vi "UHR-Fleezers Control (host) - 10.4.vi"() -> ()   [LabVIEW 2011] (continued)
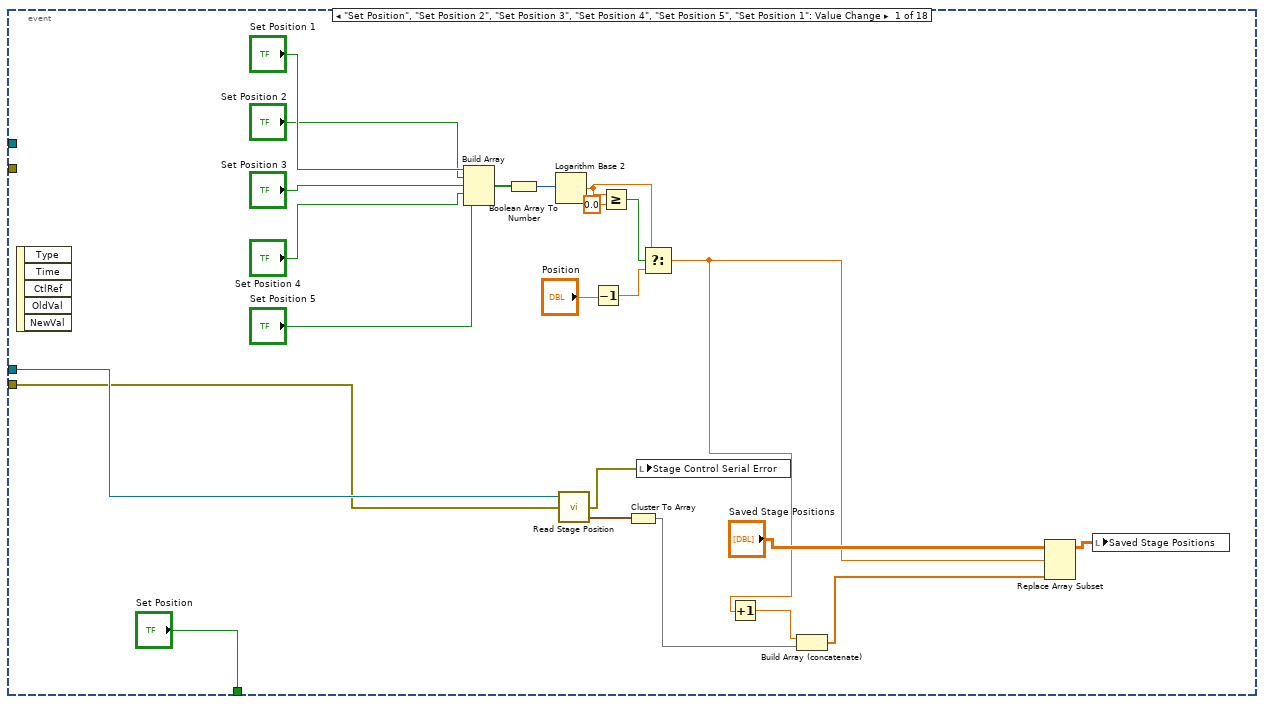
[diagram p2: hidden frame]
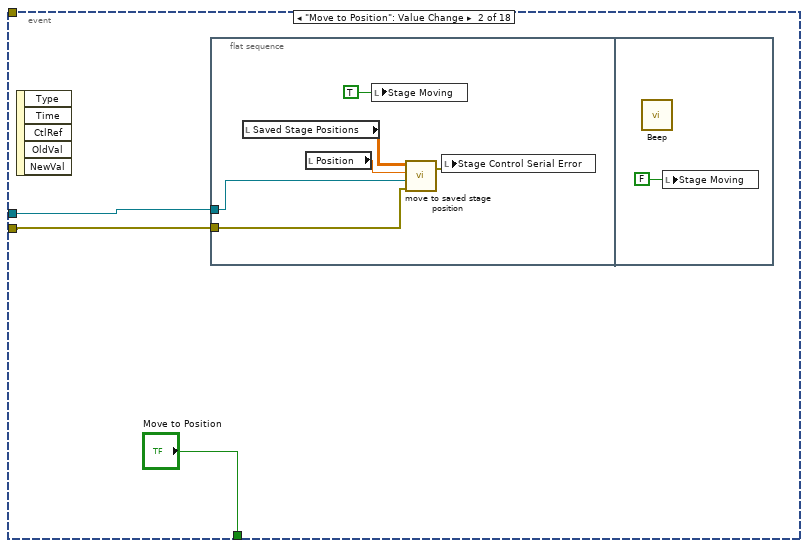
[diagram p3: hidden frame]
      tunnel: [w3040 w3060] -> w2741
      tunnel: [w3041 w3059] -> w2740
      frame False {
      }
      frame True {
        n2177 = xnode "Read/Write Control"("FPGA VI Reference In"=w3062, "error in"=w3061) -> ("FPGA VI Reference Out"=w3060:T19, "error out"=w3059:errorcluster, "GI Relative phase"=→"GI relative phase":i16, "Relative phase"=→"Relative phase (AI1)":i16, "AI Late Counter"=→"Late Counter (AI1)":u16, "GI Late Counter"=→"GI Late Counter":u16, "MCL Late Counter"=→"MCL Late Counter":u16, "MCL Relative Phase"=→"Relative Phase (MCL)":i16, "APD Acq Relative Phase"=→"APD Acq Relative Phase":i16, "APD 1 Gate Relative Phase"=→"APD 1 Gate Relative Phase":i16, "APD 2 Gate Relative Phase"=→"APD 2 Gate Relative Phase":i16, "APD Acq Late Counter"=→"APD Acq Late Counter":u16, "APD 1 Gate Late Counter"=→"APD 1 Gate Late Counter":u16, "APD 2 Gate Late Counter"=→"APD 2 Gate Late Counter":u16, "Green FB Relative Phase"=→"Relative phase (Green FB)":i16, "GI Relative phase 2"=→"GI relative phase 2":i16, "GI Late Counter 2"=→"GI Late Counter 2":u16, "Trap Pos FIFO Timeout"=→"Trap Pos FIFO Timeout":u16, "Trap AI FIFO Timeout"=→"Trap AI FIFO Timeout":u16)
      }
    }
    n2178 = call <vilib>:"Mean.vi"("X"=w2714) -> ("mean"=w2539:dbl)  [unwired: 1 out]
    "T2 X" <- w2539
    n2179 = Negate(x=w2714) -> (-x=w2715:dbl[])
    n2180 = call <vilib>:"Mean.vi"("X"=w2537) -> ("mean"=w2540:dbl)  [unwired: 1 out]
    "T1 X" <- w2540
    n2181 = Negate(x=w2539) -> (-x=w2538:dbl)
    n2182 = Bundle By Name(cluster=w2749, "Y"=w2712) -> (w2685:waveform(dbl))
    "Bead Separation" <- w2685
    n2183 = Add(x=w2537, y=w2715) -> (x+y=w2716:dbl[])
    n2184 = Add(x=w2540, y=w2538) -> (x+y=w2765:dbl)
    n2185 = Subtract(x=w2540, y=w2538) -> (x-y=→"Difference":dbl)
    n2186 = Divide(x=w2716, y=2.0) -> (x/y=→"Vec Mean of T1 T2":dbl[])
    n2187 = Divide(x=w2765, y=2.0) -> (x/y=w2718:dbl)
    "Mean" <- w2718
    n2188 = feedback-in #21("Trap Trig. Fl.") -> ()
    n2189 = feedback #21("Trap Trig. Fl.") -> (w2571:bool)
    n2190 = And(x=w2573, y=w2571) -> (x .and. y?=w2572:bool)
    n2191 = case "If have just turned off triggering" shown="True" w2572 {
      tunnel: w2553 -> [_ w2875]
      tunnel: w2552 -> [_ w2874]
      frame False {
      }
      frame True {
        w2873 = FALSE ("FPGA Trap Trig")
        n2192 = xnode "Read/Write Control"("FPGA VI Reference In"=w2875, "error in"=w2874, "FPGA Trap Trig"=w2873) -> ("FPGA VI Reference Out"=w2872:T19, "error out"=w2871:errorcluster)
        n2193 = xnode "Read/Write Control"("FPGA VI Reference In"=w2872, "error in"=w2871, "TTrig?"=w2873) -> ()  [unwired: 2 out]
        n2194 = local write "Initializing"(FALSE ("Initializing")) -> ()
        n2195 = local write "Triggered"(FALSE ("Triggered")) -> ()
        n2196 = local write "Waiting"(FALSE ("Waiting")) -> ()
      }
    }
    n2197 = Not(x=w2571) -> (.not. x?=w2584:bool)
    n2198 = And(x="Trap Trig. Fl.", y=w2584) -> (x .and. y?=w2581:bool)
    n2199 = local read "Tether"() -> (w2719:bool)
    n2200 = Or(x=w2581, y="Reinitialize") -> (x .or. y?=w2567:bool)
    n2201 = feedback #22(w2577) -> (w2582:string)
    n2202 = Select(t=w2577, s=w2581, f=w2582) -> (s? t:f=w2576:string)
    n2203 = Select(t=w2577, s="Reinitialize", f=w2576) -> (s? t:f=w2575:string)
    n2204 = feedback #23(0) -> (w2579:i32)
    n2205 = feedback #24(w2712) -> (w2711:dbl[])
    n2206 = Build Array (concatenate)(w2712, w2711) -> (w2710:dbl[])
    n2207 = case "For determining if there is a tether still" shown="True" w2719 {
      tunnel: w2718 -> [_ w2999]
      frame False {
      }
      frame True {
        n2208 = Greater?(x="Lost Tether Alarm Threshold (pN)", y=w2999) -> (0:w2997:bool)
        n2209 = case shown="True" w2997 {
          frame False {
          }
          frame True {
            w3000 = FALSE ("Value (Signaling)")
            n2210 = flat-sequence {
              frame #0 {
                # "stop only if saving"
                n2211 = local read "Saving..."() -> (w3012:bool)
                n2212 = And(x=w3012, y="TA Cancel Save?") -> (x .and. y?=w3011:bool)
                n2213 = local write "Stop Saving"(w3011) -> ()
              }
              frame #1 {
                n2214 = case shown="True" "TA Green Off?" {
                  frame False {
                  }
                  frame True {
                    w3015 = FALSE ("Fl. Triggered...")
                    n2215 = local write "Fl. Triggered..."(w3015) -> ()
                    n2216 = property on="Green Laser ON/Interlacing" class="Bool (strict)"("Val(Sgnl)"=w3015) -> ()  [unwired: 2 in, 2 out]
                  }
                }
              }
            }
            n2217 = local read "Time tether formed"() -> (w3006:timestamp)
            n2218 = Get Date/Time In Seconds() -> (seconds since 1Jan1904=w3007:timestamp)
            n2219 = Subtract(x=w3007, y=w3006) -> (x-y=w3005:dbl)
            n2220 = Number To Decimal String(number=w3005) -> (decimal integer string=w3002:string)  [unwired: 1 out]
            n2221 = local read "Messages"() -> (w3009:string)
            n2222 = call <vilib>:"Beep.vi"() -> ()  [unwired: 3 in, 9 out]
            n2223 = Concatenate Strings("Lost tether (" ("Message to add"), w3002, " s)." ("string")) -> (w3004:string)
            n2224 = local write "Tether"(FALSE ("Tether")) -> ()
            n2225 = call "Update messages.vi"("Message to add"=w3004, "Old message string"=w3009) -> ("New message string"=w3008:string)
            n2226 = local write "Messages"(w3008) -> ()
            n2227 = local write "Dip for Protein"(w3000) -> ()
            n2228 = property on="Trap Pos. FB ON" class="Bool (strict)"("Val(Sgnl)"=w3000) -> ()  [unwired: 2 in, 2 out]
            n2229 = property on="Trap Trig. Fl." class="Bool (strict)"("Val(Sgnl)"=w3000) -> ()  [unwired: 2 in, 2 out]
          }
        }
      }
    }
    n2230 = case "For triggering actions based on the trap position (e.g., turning the excitation laser on if trap under feedback moves so far)" shown="True" "Trap Trig. Fl." {
      tunnel: w2562 -> [_ w2888]
      tunnel: w2575 -> [_ w2887]
      tunnel: ["" ("t") w2886] -> w2583
      tunnel: w2567 -> [_ w2885]
      tunnel: [0 ("t") w2884] -> w2580
      tunnel: w2579 -> [_ w2883]
      tunnel: w2553 -> [_ w2882]
      tunnel: w2552 -> [_ w2881]
      frame False {
      }
      frame True {
        n2231 = case shown="\"Initialize\", Default" w2887 {
          tunnel: w2888 -> [w2905 _ _ w2953]
          tunnel: [w2902 w2934 "" ("t") w2956] -> w2886
          tunnel: w2885 -> [_ _ _ w2944]
          tunnel: [w2901 w2931 0 ("t") w2945] -> w2884
          tunnel: w2883 -> [_ w2933 _ w2951]
          tunnel: w2882 -> [w2890 w2928 _ w2947]
          tunnel: w2881 -> [w2889 w2927 _ w2946]
          frame "Wait for trigger" {
            n2232 = local read "Trap Trig. (FPGA)"() -> (w2893:bool)
            n2233 = Subtract(x=w2905, y="Mean T1 Position\nto compare (nm)") -> (x-y=w2898:dbl[])
            n2234 = call <vilib>:"Std Deviation and Variance.vi"("X"=w2898) -> ("mean"=→"mean":dbl, "standard deviation"=→"standard\ndeviation":dbl)  [unwired: 1 in, 1 out]
            n2235 = Array Max & Min(array=w2898) -> (max value=→"max value":dbl, min value=→"min value":dbl)  [unwired: 2 out]
            n2236 = Greater?(x=w2898, y="Threshold (nm)") -> (0:w2908:bool[])
            n2237 = case shown="True" w2893 {
              tunnel: w2890 -> [_ w2914]
              tunnel: w2889 -> [_ w2913]
              tunnel: [FALSE ("TTrig?") w2912] -> w2896
              frame False {
              }
              frame True {
                n2238 = xnode "Read/Write Control"("FPGA VI Reference In"=w2914, "error in"=w2913) -> ("TTrig?"=w2912:bool)  [unwired: 2 out]
              }
            }
            n2239 = Or Array Elements(Boolean array=w2908) -> (logical OR=w2895:bool)
            n2240 = Select(t=w2896, s=w2893, f=w2895) -> (s? t:f=w2894:bool)
            n2241 = Not(x=w2893) -> (.not. x?=w2892:bool)
            n2242 = And(x=w2894, y=w2892) -> (x .and. y?=w2891:bool)
            n2243 = Select(t="Triggered", s=w2894, f="Wait for trigger") -> (s? t:f=w2902:string)
            n2244 = case shown="True" w2894 {
              tunnel: [0 0] -> w2901
              tunnel: w2890 -> [_ w2919]
              tunnel: w2889 -> [_ w2918]
              frame False {
                "Waiting" <- TRUE ("Waiting")
              }
              frame True {
                n2245 = xnode "Read/Write Control"("FPGA VI Reference In"=w2919, "error in"=w2918, "TTrig?"=FALSE) -> ()  [unwired: 2 out]
                n2246 = local read "Messages"() -> (w2922:string)
                n2247 = call <vilib>:"Beep.vi"() -> ()  [unwired: 12 in]
                n2248 = call "Update messages.vi"("Message to add"="Unwinding trigger.", "Old message string"=w2922) -> ("New message string"=w2923:string)
                n2249 = local write "Messages"(w2923) -> ()
                n2250 = local write "Waiting"(FALSE ("Waiting")) -> ()
                "Triggered" <- TRUE ("Triggered")
              }
            }
            n2251 = case "Only need to turn on laser if host triggered" shown="True" w2891 {
              frame False {
              }
              frame True {
                n2252 = property on="Green Laser ON/Interlacing" class="Bool (strict)"("Val(Sgnl)"=TRUE ("Value (Signaling)")) -> ()  [unwired: 2 in, 2 out]
              }
            }
          }
          frame "Triggered" {
            n2253 = local read "Trap Trig. (FPGA)"() -> (w2930:bool)
            n2254 = Increment(x=w2933) -> (x+1=w2931:i32)
            n2255 = Greater Or Equal?(x=w2931, y="Fl. ON time (n)") -> (x >= y?=w2929:bool)
            n2256 = Select(t="Wait for trigger", s=w2929, f="Triggered" ("t")) -> (s? t:f=w2934:string)
            n2257 = And(x=w2929, y=w2930) -> (x .and. y?=w2926:bool)
            n2258 = case shown="True" w2926 {
              tunnel: w2928 -> [_ w2938]
              tunnel: w2927 -> [_ w2937]
              frame False {
              }
              frame True {
                n2259 = xnode "Read/Write Control"("FPGA VI Reference In"=w2938, "error in"=w2937, "FPGA Trap Trig"=TRUE) -> ()  [unwired: 2 out]
              }
            }
            n2260 = case shown="True" w2929 {
              frame False {
              }
              frame True {
                w2940 = FALSE ("Value (Signaling)")
                n2261 = local write "Triggered"(w2940) -> ()
                n2262 = local write "Waiting"(TRUE ("Waiting")) -> ()
                n2263 = property on="Green Laser ON/Interlacing" class="Bool (strict)"("Val(Sgnl)"=w2940) -> ()  [unwired: 2 in, 2 out]
              }
            }
          }
          frame "Do nothing" {
          }
          frame "Initialize", Default {
            n2264 = Increment(x=w2951) -> (x+1=w2955:i32)
            n2265 = Select(t=1, s=w2944, f=w2955) -> (s? t:f=w2945:i32)
            n2266 = feedback #25(w2953) -> (w2959:dbl[])
            n2267 = Build Array (concatenate)(w2953, w2959) -> (w2952:dbl[])
            n2268 = Greater Or Equal?(x=w2945, y="Wait to get offset (n)") -> (x >= y?=w2948:bool)
            n2269 = Select(t=w2953, s=w2944, f=w2952) -> (s? t:f=w2954:dbl[])
            n2270 = feedback-in #25(w2954) -> ()
            n2271 = call <vilib>:"Mean.vi"("X"=w2954) -> ("mean"=w2949:dbl)  [unwired: 1 out]
            n2272 = local write "Mean T1 Position\nto compare (nm)"(w2949) -> ()
            n2273 = case shown="True" w2944 {
              tunnel: w2947 -> [_ w2965]
              tunnel: w2946 -> [_ w2964]
              frame False {
              }
              frame True {
                w2961 = FALSE ("FPGA Trap Trig")
                n2274 = xnode "Read/Write Control"("FPGA VI Reference In"=w2965, "error in"=w2964, "FPGA Trap Trig"=w2961) -> ("FPGA VI Reference Out"=w2963:T19, "error out"=w2962:errorcluster)
                n2275 = xnode "Read/Write Control"("FPGA VI Reference In"=w2963, "error in"=w2962, "TTrig?"=w2961) -> ()  [unwired: 2 out]
              }
            }
            n2276 = Select(t="Wait for trigger", s=w2948, f="Initialize") -> (s? t:f=w2956:string)
            n2277 = case shown="True" w2948 {
              tunnel: w2949 -> [_ w2968]
              tunnel: w2947 -> [_ w2977]
              tunnel: w2946 -> [_ w2976]
              frame False {
                n2278 = local write "Waiting"(FALSE ("Waiting")) -> ()
                "Initializing" <- TRUE ("Initializing")
              }
              frame True {
                n2279 = local read "Threshold (nm)"() -> (w2980:dbl)
                n2280 = local read "AOM X Cal (nm/MHz)"() -> (w2979:dbl)
                n2281 = Add(x=w2968, y=w2980) -> (x+y=w2981:dbl)
                n2282 = Divide(x=w2981, y=w2979) -> (x/y=w2978:dbl)
                n2283 = call "IR AOM freq to word.vi"("Frequency In (MHz)"=w2978) -> ("Frequency Word Out (double)"=w2975:dbl)
                n2284 = local write "Initializing"(FALSE ("Initializing")) -> ()
                n2285 = local write "Waiting"(TRUE ("Waiting")) -> ()
                n2286 = To Quad Integer(1:w2975) -> (0:w2974:i64)
                n2287 = xnode "Read/Write Control"("FPGA VI Reference In"=w2977, "error in"=w2976, "FPGA TTrig Thresh"=w2974) -> ("FPGA VI Reference Out"=w2971:T19, "error out"=w2970:errorcluster)
                n2288 = xnode "Read/Write Control"("FPGA VI Reference In"=w2971, "error in"=w2970, "FPGA Trap Trig"=TRUE) -> ()  [unwired: 2 out]
              }
            }
          }
        }
      }
    }
    n2289 = feedback-in #22(w2583) -> ()
    n2290 = feedback-in #23(w2580) -> ()
    n2291 = Split 1D Array(array=w2710, index=w2597) -> (first subarray=w2707:dbl[])  [unwired: 1 out]
    n2292 = feedback-in #24(w2707) -> ()
    n2293 = call <vilib>:"Mean.vi"("X"=w2707) -> ("mean"=w2706:dbl)  [unwired: 1 out]
    "Bead Mean (nm)" <- w2706
    n2294 = Subtract(x=w2707, y=w2706) -> (x-y=w2705:dbl[])
    n2295 = Square(x=w2705) -> (x^2=w2704:dbl[])
    n2296 = call <vilib>:"Mean.vi"("X"=w2704) -> ("mean"=w2703:dbl)  [unwired: 1 out]
    n2297 = Square Root(x=w2703) -> (sqrt(x)=w2702:dbl)
    n2298 = Multiply(x=10.0, y=w2702) -> (x*y=→"RMS (Ang)":dbl)
    n2299 = xnode "Read/Write Control"("FPGA VI Reference In"=w2741, "error in"=w2740) -> ("FPGA VI Reference Out"=w2565:T19, "error out"=w2564:errorcluster, "AI2 Y Sum Set 1"=w2849:i16, "AI2 Y Sum Set 2"=w2848:i16, "AI1 X Set 1"=w2629:fxp<+/-,16,1>, "AI1 X Set 2"=w2628:fxp<+/-,16,1>, "Trap Pos FB Int Signal"=→"Trap Pos FB Int Signal":fxp<+/-,24,9>, "Trap Pos FB Int-Norm Signal"=→"Trap Pos FB Int-Norm Signal":fxp<+/-,16,1>, "Trap Pos FB Action"=w2622:i64, "Scanning"=→"AOD Scanning":bool, "Scan I"=→"AOD Scan I":u64, "Scanning MCL"=w2851:bool, "Scan I (MCL)"=→"MCL Scan I":u64, "Green FB Signals"=w2788:T46, "TTrig Sig"=w2551:i64, "TTrig Fin Thresh"=w2547:i64)
    "MCL Scanning" <- w2851
    "Trap Pos FB Action" <- w2622
    n2300 = local read "FB Trig Integrate"() -> (w2545:u32)
    n2301 = Divide(x=w2551, y=w2545) -> (x/y=w2544:dbl)
    "TTrig Sig (Int)" <- w2544
    n2302 = Divide(x=w2547, y=w2545) -> (x/y=w2542:dbl)
    "TTrig Fin Thresh (Int)" <- w2542
    n2303 = local read "AOM X Cal (nm/MHz)"() -> (w2550:dbl)
    n2304 = local read "AI2 (V)"() -> (w2850:cluster{"Set 1":dbl, "Set 2":dbl})
    n2305 = Bundle By Name(cluster=w2850, "Set 1"=w2849, "Set 2"=w2848) -> (w2846:cluster{"Set 1":dbl, "Set 2":dbl})
    n2306 = Divide(x=w2622, y=327.67) -> (x/y=→"Action (%)":dbl)
    n2307 = local read "Trap X (AI1)"() -> (w2642:T10)
    n2308 = call "IR AOM word double to freq.vi"("Frequency Word In (double)"=w2542) -> ("Frequency Out (MHz)"=w2541:dbl)
    n2309 = call "IR AOM word double to freq.vi"("Frequency Word In (double)"=w2544) -> ("Frequency Out (MHz)"=w2543:dbl)
    n2310 = Divide(x=w2846, y=3276.7) -> (x/y=w2845:cluster{"Set 1":dbl, "Set 2":dbl})
    n2311 = Multiply(x=w2543, y=w2550) -> (x*y=w2549:dbl)
    "TTrig Sig (nm)" <- w2549
    n2312 = Multiply(x=w2541, y=w2550) -> (x*y=w2548:dbl)
    "TTrig Fin Thresh (nm)" <- w2548
    n2313 = local write "AI2 (V)"(w2845) -> ()
    n2314 = Bundle(cluster=w2642, "Trap 1"=w2629, "Trap 2"=w2628) -> (→"Trap X (AI1)":T10)
    n2315 = Bundle(w2549, w2548) -> (→"TTrig":cluster{dbl, dbl})  [unwired: 1 in]
    n2316 = Divide(x=w2788, y=3276.7) -> (x/y=w2784:T47)
    n2317 = Unbundle By Name(w2784) -> ("Green FB Ch 0"=w2787:dbl, "Green FB Ch 1"=w2786:dbl, "Green FB Ch 2"=w2785:dbl)
    n2318 = Divide(x=w2787, y=w2785) -> (x/y=w2783:dbl)
    n2319 = Divide(x=w2786, y=w2785) -> (x/y=w2782:dbl)
    n2320 = flat-sequence "To save data" {
      tunnel: [w3836] -> w2869
      tunnel: [w3837] -> w2868
      tunnel: w2819 -> [w3830]
      tunnel: w2570 -> [w3834]
      tunnel: ["Save Calibration"] -> w2842
      tunnel: w2839 -> [w3833]
      tunnel: [w3826] -> w2838
      tunnel: [w3823] -> w2837
      tunnel: [w3820] -> w2836
      tunnel: w2818 -> [w3822]
      tunnel: w2723 -> [w3816]
      tunnel: [w3816] -> w2722
      tunnel: ["Start Saving"] -> w2687
      tunnel: [w3810] -> w2610
      tunnel: [w3809] -> w2609
      tunnel: w2869 -> [w4071]
      tunnel: w2868 -> [w4070]
      tunnel: w2611 -> [w4069]
      tunnel: w2842 -> [w4068]
      tunnel: w2838 -> [w4066]
      tunnel: w2837 -> [w4065]
      tunnel: w2836 -> [w4064]
      tunnel: w2696 -> [w4063]
      tunnel: w2733 -> [w4062]
      tunnel: w2722 -> [w4061]
      tunnel: w2687 -> [w4060]
      tunnel: w2685 -> [w4059]
      tunnel: w2661 -> [w4058]
      tunnel: w2610 -> [w4057]
      tunnel: w2609 -> [w4056]
      tunnel: w2608 -> [w4055]
      frame #0 {
        n2321 = Or(x="Save N Sets", y="Start Saving") -> (x .or. y?=w3817:bool)
        n2322 = To Double Precision Float(number=w3833) -> (double precision float=w3827:dbl)
        n2323 = Build Array(w3817, "Save Calibration", w3830, w3822) -> (w3832:bool[])
        n2324 = Compound Arithmetic op=OR("Save Calibration", w3830, w3817, w3822) -> (w3835:bool)
        n2325 = Boolean Array To Number(Boolean array=w3832) -> (number=w3829:u32)
        n2326 = feedback #26(FALSE ("Save APD Data\nwith Trap Data")) -> (w3811:bool)
        n2327 = feedback #27(refnum<k0> refnum) -> (w3838:refnum<file>)
        n2328 = feedback #28(refnum<k0> refnum) -> (w3813:refnum<file>)
        n2329 = feedback #29(FALSE ("Save APD Data\nwith Trap Data")) -> (w3821:bool)
        n2330 = feedback #30(refnum<k0> refnum) -> (w3824:refnum<file>)
        n2331 = feedback #31(0) -> (w3840:i32)
        n2332 = feedback #32() -> (w3828:u32)  [unwired: 1 out]
        n2333 = case shown="True" w3835 {
          tunnel: [w3847 1] -> w3836
          tunnel: w3840 -> [w3849 _]
          tunnel: [w3848 w3867] -> w3837
          tunnel: w3838 -> [w3848 _]
          tunnel: w3834 -> [_ w3887]
          tunnel: w3827 -> [_ w3885]
          tunnel: w3829 -> [_ w3888]
          tunnel: [w3846 w3866] -> w3826
          tunnel: w3828 -> [w3846 _]
          tunnel: [w3845 w3864] -> w3823
          tunnel: w3824 -> [w3845 _]
          tunnel: [w3844 w3863] -> w3820
          tunnel: w3821 -> [w3844 _]
          tunnel: "Start Saving" -> [_ w3861]
          tunnel: w3816 -> [_ w3860]
          tunnel: [w3843 w3851] -> w3809
          tunnel: w3813 -> [w3843 _]
          tunnel: [w3842 w3850] -> w3810
          tunnel: w3811 -> [w3842 _]
          frame False {
            n2334 = Increment(x=w3849) -> (x+1=w3847:i32)
          }
          frame True {
            w3857 = FALSE ("Start Saving")
            w3862 = 9.0  # File Version
            w3870 = FALSE ("prepend array or string size? (T)")
            w3868 = T24."big-endian, network order" ("byte order (0:big-endian, network order)")
            n2335 = local read "BD 1 Frequency 1 (MHz)"() -> (w3884:dbl)
            n2336 = local read "BD 2 Frequency 1 (MHz)"() -> (w3883:dbl)
            n2337 = local read "BD 1 Frequency 2 (MHz)"() -> (w3882:dbl)
            n2338 = local read "BD 2 Frequency 2 (MHz)"() -> (w3881:dbl)
            n2339 = local read "BD 1 Frequency 3 (MHz)"() -> (w3880:dbl)
            n2340 = local read "BD 2 Frequency 3 (MHz)"() -> (w3879:dbl)
            n2341 = Array Size(array=w3860) -> (size(s)=w3859:i32)
            n2342 = To Double Precision Float(number=w3859) -> (double precision float=w3858:dbl)
            n2343 = local write "Save Calibration"(w3857) -> ()
            n2344 = local write "Start Saving"(w3857) -> ()
            n2345 = Build Array("Save APD Data\nwith Trap Data", "Save Trap Pos. Data") -> (w3854:bool[])
            n2346 = Boolean Array To Number(Boolean array=w3854) -> (number=w3853:u32)
            n2347 = Build Array(w3884, w3883, w3882, w3881, w3880, w3879) -> (w3878:dbl[])
            n2348 = case shown="4" w3888 {
              tunnel: w3887 -> [w3959 w3979 w3995 w4033]
              tunnel: w3858 -> [w3964 w3986 w4015 w4052]
              tunnel: w3885 -> [w3963 w3985 w4014 w4051]
              tunnel: [w3960 w3981 w4006 w4043] -> w3876
              tunnel: [w3951 "Cal sets to save" w3996 w4034] -> w3866
              tunnel: w3878 -> [w3961 w3982 w4008 w4045]
              tunnel: "Save APD Data\nwith Trap Data" -> [w3958 _ w3992 w4031]
              tunnel: [w3958 w3973 w3992 w4031] -> w3863
              tunnel: w3862 -> [w3954 w3974 w3990 w4029]
              tunnel: w3861 -> [w3953 _ _ _]
              tunnel: [w3944 w3973 w3989 w4019] -> w3850
              tunnel: "Save Trap Pos. Data" -> [w3944 _ w3989 w4019]
              tunnel: w3853 -> [w3943 _ w3988 w4018]
              frame 1, Default {
                # "timeseries"
                n2349 = case shown="True" "Profile" {
                  tunnel: [w3967 w3971] -> w3948
                  tunnel: [w3967 w3970] -> w3947
                  tunnel: [w3967 w3969] -> w3946
                  tunnel: [w3967 w3968] -> w3945
                  frame False {
                    w3967 = 0.0 ("f")
                  }
                  frame True {
                    n2350 = local read "Current Position"() -> (w3972:cluster{dbl, dbl, dbl})
                    n2351 = local read "Y change (mm)"() -> (w3968:dbl)
                    n2352 = Unbundle(w3972) -> (w3971:dbl, w3970:dbl, w3969:dbl)
                  }
                }
                n2353 = local read "Save ave N"() -> (w3966:dbl)
                n2354 = Multiply(x=w3966, y=w3959) -> (x*y=w3965:dbl)
                n2355 = To Double Precision Float(number=w3943) -> (double precision float=w3957:dbl)
                n2356 = Build Array(w3954, w3959, w3965, w3964, w3963, 0.0 ("f")) -> (w3962:dbl[])
                n2357 = Build Array(w3957, w3948, w3947, w3946, w3945) -> (w3955:dbl[])
                n2358 = Select(t=u32 4000000000, s=w3953, f="N sets to save") -> (s? t:f=w3951:u32)
                n2359 = Build Array (concatenate)(w3962, w3961, w3955) -> (w3960:dbl[])
              }
              frame 2 {
                w3976 = 0.0 ("f")
                w3973 = FALSE ("Save APD Data\nwith Trap Data")
                # "calibration"
                n2360 = Boolean To (0,1)(Boolean=w3973) -> (0, 1=w3978:i16)
                n2361 = To Double Precision Float(number=w3978) -> (double precision float=w3977:dbl)
                n2362 = Build Array(w3977, w3976, w3976, w3976, w3976) -> (w3975:dbl[])
                n2363 = Build Array(w3974, w3979, w3979, w3986, w3985, 1.0 ("t")) -> (w3983:dbl[])
                n2364 = Build Array (concatenate)(w3983, w3982, w3975) -> (w3981:dbl[])
                "Calibrating Trap..." <- TRUE ("Calibrating...")
              }
              frame 4 {
                w3993 = 0.0 ("f")
                # "scan dir (x/y = 0/1)"
                # "cycles/step"
                # "n scans (f/b)"
                # "steps"
                # "freq. range"
                # "AOD raster scan"
                n2365 = local read "Number of F/B Scans (AOD)"() -> (w4000:u16)
                n2366 = local read "Cycles/step (AOD)"() -> (w4002:u64)
                n2367 = local read "Scan Range (MHz)"() -> (w4005:dbl)
                n2368 = local read "Scan steps (AOD)"() -> (w4004:u64)
                n2369 = local read "Scan BD"() -> (w4012:bool)
                n2370 = local read "Save ave N"() -> (w4017:dbl)
                n2371 = Boolean To (0,1)(Boolean=w4012) -> (0, 1=w4011:i16)
                n2372 = To Double Precision Float(number=w4000) -> (double precision float=w3999:dbl)
                n2373 = To Double Precision Float(number=w4004) -> (double precision float=w4003:dbl)
                n2374 = To Double Precision Float(number=w4002) -> (double precision float=w4001:dbl)
                n2375 = To Double Precision Float(number=w4011) -> (double precision float=w4010:dbl)
                n2376 = Multiply(x=w4017, y=w3995) -> (x*y=w4016:dbl)
                n2377 = To Double Precision Float(number=w3988) -> (double precision float=w3994:dbl)
                n2378 = Build Array(w3994, w3993, w3993, w3993, w3993) -> (w3991:dbl[])
                n2379 = local read "N sets should be saved"() -> (w3997:dbl)
                n2380 = Build Array(w4010, w4005, w4003, w4001, w3999) -> (w4007:dbl[])
                n2381 = Build Array(w3990, w3995, w4016, w4015, w4014, 2.0 ("t")) -> (w4009:dbl[])
                n2382 = Round Toward +Infinity(x=w3997) -> (ceil(x): smallest int >= x=w3998:dbl)
                n2383 = Build Array (concatenate)(w4009, w4008, w3991, w4007) -> (w4006:dbl[])
                n2384 = To Unsigned Long Integer(number=w3998) -> (unsigned 32bit integer=w3996:u32)
              }
              frame 8 {
                w4026 = 0.0 ("f")
                # "MCL raster scan"
                n2385 = local read "Number of scans (MCL)"() -> (w4021:u64)
                n2386 = local read "Scan lines (y)"() -> (w4020:u64)
                n2387 = local read "2D or 1D Scan"() -> (w4023:bool)
                n2388 = local read "Scan Range (V)\n(of steps)"() -> (w4042:dbl)
                n2389 = local read "Fast Scan Dir"() -> (w4049:bool)
                n2390 = local read "Cycles/step (MCL)"() -> (w4039:u64)
                n2391 = local read "Scan steps (MCL)"() -> (w4041:u64)
                n2392 = Select(t=w4020, s=w4023, f=w4021) -> (s? t:f=w4022:u64)
                n2393 = Boolean To (0,1)(Boolean=w4023) -> (0, 1=w4025:i16)
                n2394 = local read "Save ave N"() -> (w4054:dbl)
                n2395 = local read "Initial X"() -> (w4028:dbl)
                n2396 = local read "Initial Y"() -> (w4027:dbl)
                n2397 = To Double Precision Float(number=w4025) -> (double precision float=w4024:dbl)
                n2398 = Boolean To (0,1)(Boolean=w4049) -> (0, 1=w4048:i16)
                n2399 = To Double Precision Float(number=w4022) -> (double precision float=w4037:dbl)
                n2400 = To Double Precision Float(number=w4041) -> (double precision float=w4040:dbl)
                n2401 = To Double Precision Float(number=w4039) -> (double precision float=w4038:dbl)
                n2402 = To Double Precision Float(number=w4048) -> (double precision float=w4047:dbl)
                n2403 = Multiply(x=w4054, y=w4033) -> (x*y=w4053:dbl)
                n2404 = To Double Precision Float(number=w4018) -> (double precision float=w4032:dbl)
                n2405 = local read "N sets should be saved (MCL)"() -> (w4035:dbl)
                n2406 = Build Array(w4032, w4024, w4026, w4026, w4026) -> (w4030:dbl[])
                n2407 = Build Array(w4047, w4042, w4040, w4038, w4037, w4028, w4027) -> (w4044:dbl[])
                n2408 = Build Array(w4029, w4033, w4053, w4052, w4051, 3.0 ("t")) -> (w4046:dbl[])
                n2409 = Round Toward +Infinity(x=w4035) -> (ceil(x): smallest int >= x=w4036:dbl)
                n2410 = Build Array (concatenate)(w4046, w4045, w4030, w4044) -> (w4043:dbl[])
                n2411 = To Unsigned Long Integer(number=w4036) -> (unsigned 32bit integer=w4034:u32)
              }
            }
            n2412 = local read "Index"() -> (w3893:dbl)
            n2413 = call "Create new save file.vi"("Insert"="", "Ext"=".dat", "Index In"=w3893) -> ("Path Out"=w3852:path, "Index Out"=w3865:dbl)
            n2414 = local write "Save file name"(w3852) -> ()
            n2415 = local write "Index"(w3865) -> ()
            n2416 = local write "Save index"(w3865) -> ()
            n2417 = Array Size(array=w3876) -> (size(s)=w3877:i32)
            n2418 = Open/Create/Replace File(file path (use dialog)=w3852, operation (0:open)=T25."create", access (0:read/write)=enum16{"read/write", "read-only", "write-only"}."write-only") -> (refnum out=w3890:refnum<file>)  [unwired: 1 in, 4 out]
            n2419 = local write "Saving..."(TRUE ("Saving...")) -> ()
            n2420 = To Double Precision Float(number=w3877) -> (double precision float=w3875:dbl)
            n2421 = String Length(string="Comment (data description)") -> (length=w3873:i32)
            n2422 = To Double Precision Float(number=w3873) -> (double precision float=w3872:dbl)
            n2423 = Deny Access(7:w3890) -> (3:w3889:refnum<file>)  [unwired: 1 in, 2 out]
            n2424 = Build Array (concatenate)(w3875, w3876, w3872) -> (w3874:dbl[])
            n2425 = case "If fluorescence data to be saved" shown="True" w3863 {
              tunnel: w3852 -> [_ w3942]
              tunnel: [refnum<k0> refnum w3922] -> w3864
              frame False {
              }
              frame True {
                w3921 = 0.0
                n2426 = local read "APD Integration Time (s)"() -> (w3927:dbl)
                n2427 = local read "N APD Samp/step"() -> (w3920:dbl)
                n2428 = Path To String(path=w3942) -> (string=w3941:string)
                n2429 = String Length(string=w3941) -> (length=w3940:i32)
                n2430 = Subtract(x=w3940, y=4) -> (x-y=w3938:i32)
                n2431 = String Subset(string=w3941, length (rest)=w3938) -> (substring=w3937:string)  [unwired: 1 out]
                n2432 = Build Array(w3927, w3920, w3921, w3921, w3921, w3921, w3921, w3921) -> (w3924:dbl[])
                n2433 = Concatenate Strings(w3937, "_fl.dat" ("string")) -> (w3935:string)
                n2434 = Array Size(array=w3924) -> (size(s)=w3926:i32)
                n2435 = String To Path(string=w3935) -> (path=w3931:path)
                n2436 = Open/Create/Replace File(file path (use dialog)=w3931, operation (0:open)=T25."create", access (0:read/write)=enum16{"read/write", "read-only", "write-only"}."write-only") -> (refnum out=w3932:refnum<file>)  [unwired: 1 in, 4 out]
                n2437 = Deny Access(7:w3932) -> (3:w3928:refnum<file>)  [unwired: 1 in, 2 out]
                n2438 = To Double Precision Float(number=w3926) -> (double precision float=w3925:dbl)
                n2439 = Build Array (concatenate)(w3925, w3924) -> (w3923:dbl[])
                n2440 = Write to Binary File(file (use dialog)=w3928, data=w3923, 5:FALSE ("prepend array or string size? (T)"), 9:T24."big-endian, network order" ("byte order (0:big-endian, network order)")) -> (refnum out=w3922:refnum<file>)  [unwired: 1 in, 3 out]
              }
            }
            n2441 = case shown="True" w3850 {
              tunnel: w3852 -> [_ w3904]
              tunnel: [refnum<k0> refnum w3903] -> w3851
              frame False {
              }
              frame True {
                w3899 = 0.0 ("element")
                n2442 = Path To String(path=w3904) -> (string=w3918:string)
                n2443 = Build Array(w3899, w3899, w3899, w3899, w3899, w3899, w3899, w3899) -> (w3900:dbl[])
                n2444 = String Length(string=w3918) -> (length=w3917:i32)
                n2445 = Subtract(x=w3917, y=4) -> (x-y=w3915:i32)
                n2446 = Array Size(array=w3900) -> (size(s)=w3902:i32)
                n2447 = String Subset(string=w3918, length (rest)=w3915) -> (substring=w3914:string)  [unwired: 1 out]
                n2448 = To Double Precision Float(number=w3902) -> (double precision float=w3901:dbl)
                n2449 = Concatenate Strings(w3914, "_pos.dat" ("string")) -> (w3912:string)
                n2450 = Build Array (concatenate)(w3901, w3900) -> (w3898:dbl[])
                n2451 = String To Path(string=w3912) -> (path=w3908:path)
                n2452 = Open/Create/Replace File(file path (use dialog)=w3908, operation (0:open)=T25."create", access (0:read/write)=enum16{"read/write", "read-only", "write-only"}."write-only") -> (refnum out=w3909:refnum<file>)  [unwired: 1 in, 4 out]
                n2453 = Deny Access(7:w3909) -> (3:w3905:refnum<file>)  [unwired: 1 in, 2 out]
                n2454 = Write to Binary File(file (use dialog)=w3905, data=w3898, 5:FALSE ("prepend array or string size? (T)"), 9:T24."big-endian, network order" ("byte order (0:big-endian, network order)")) -> (refnum out=w3903:refnum<file>)  [unwired: 1 in, 3 out]
              }
            }
            n2455 = Write to Binary File(file (use dialog)=w3889, data=w3874, 5:w3870, 9:w3868) -> (refnum out=w3871:refnum<file>)  [unwired: 1 in, 3 out]
            n2456 = Write to Binary File(file (use dialog)=w3871, data="Comment (data description)", 5:w3870, 9:w3868) -> (refnum out=w3867:refnum<file>)  [unwired: 1 in, 3 out]
          }
        }
        n2457 = feedback-in #26(w3810) -> ()
        n2458 = feedback-in #27(w3837) -> ()
        n2459 = feedback-in #28(w3809) -> ()
        n2460 = feedback-in #29(w3820) -> ()
        n2461 = feedback-in #30(w3823) -> ()
        n2462 = feedback-in #31(w3836) -> ()
        n2463 = feedback-in #32(w3826) -> ()
      }
      frame #1 {
        n2464 = local read "Saving..."() -> (w4067:bool)
        n2465 = case shown="True" w4067 {
          tunnel: w4071 -> [_ w4081]
          tunnel: w4070 -> [_ w4095]
          tunnel: w4069 -> [_ w4091]
          tunnel: w4068 -> [_ w4090]
          tunnel: w4066 -> [_ w4089]
          tunnel: w4065 -> [_ w4084]
          tunnel: w4064 -> [_ w4083]
          tunnel: w4063 -> [_ w4082]
          tunnel: w4062 -> [_ w4080]
          tunnel: w4061 -> [_ w4078]
          tunnel: w4060 -> [_ w4077]
          tunnel: w4059 -> [_ w4076]
          tunnel: w4058 -> [_ w4075]
          tunnel: w4057 -> [_ w4074]
          tunnel: w4056 -> [_ w4073]
          tunnel: w4055 -> [_ w4072]
          frame False {
          }
          frame True {
            n2466 = Multiply(x=w4081, y=w4080) -> (x*y=→"Time (s)":dbl)
            n2467 = Less Or Equal?(x=w4081, y=w4089) -> (x <= y?=w4093:bool)
            n2468 = Or(x="Stop Saving", y="Abort save 2") -> (x .or. y?=w4085:bool)
            n2469 = Not(x=w4085) -> (.not. x?=w4094:bool)
            n2470 = And(x=w4093, y=w4094) -> (x .and. y?=w4092:bool)
            n2471 = case shown="True" w4092 {
              tunnel: w4095 -> [w4102 w4170]
              tunnel: [0.0 w4173] -> w4088
              tunnel: w4081 -> [_ w4171]
              tunnel: w4089 -> [_ w4172]
              tunnel: w4091 -> [_ w4167]
              tunnel: w4090 -> [_ _]
              tunnel: w4084 -> [w4100 w4160]
              tunnel: w4083 -> [w4099 w4161]
              tunnel: w4082 -> [_ w4159]
              tunnel: w4078 -> [_ w4158]
              tunnel: w4077 -> [_ w4112]
              tunnel: w4076 -> [_ w4151]
              tunnel: w4075 -> [_ w4129]
              tunnel: w4074 -> [w4096 w4110]
              tunnel: w4073 -> [w4097 w4109]
              tunnel: w4072 -> [_ w4106]
              frame False {
                w4098 = FALSE
                n2472 = Close File(refnum=w4102) -> ()  [unwired: 1 in, 2 out]
                n2473 = case shown="True" w4099 {
                  tunnel: w4100 -> [_ w4104]
                  frame False {
                  }
                  frame True {
                    n2474 = Close File(refnum=w4104) -> ()  [unwired: 1 in, 2 out]
                  }
                }
                n2475 = case shown="True" w4096 {
                  tunnel: w4097 -> [_ w4103]
                  frame False {
                  }
                  frame True {
                    n2476 = Close File(refnum=w4103) -> ()  [unwired: 1 in, 2 out]
                  }
                }
                n2477 = local write "Raster Scanning..."(w4098) -> ()
                n2478 = local write "Calibrating Trap..."(w4098) -> ()
                n2479 = call <vilib>:"Beep.vi"() -> ()  [unwired: 3 in, 9 out]
                n2480 = local write "Stop Saving"(w4098) -> ()
                "Saving..." <- w4098
              }
              frame True {
                n2481 = local read "Calibrating Trap..."() -> (w4162:bool)
                n2482 = case "Write fl. data" shown="True" w4161 {
                  tunnel: w4160 -> [_ w4196]
                  tunnel: w4159 -> [_ w4195]
                  frame False {
                  }
                  frame True {
                    n2483 = Write to Binary File(file (use dialog)=w4196, data=w4195, 5:FALSE ("prepend array or string size? (T)"), 9:T24."big-endian, network order" ("byte order (0:big-endian, network order)")) -> ()  [unwired: 1 in, 4 out]
                  }
                }
                n2484 = Greater?(x="Save ave N", y=1.0) -> (0:w4165:bool)
                n2485 = Not(x=w4162) -> (.not. x?=w4164:bool)
                n2486 = And(x=w4164, y=w4165) -> (x .and. y?=w4107:bool)
                n2487 = case shown="True" w4107 {
                  tunnel: w4106 -> [w4176 w4187]
                  tunnel: [w4176 w4179] -> w4105
                  tunnel: "Save ave N" -> [_ w4180]
                  frame False {
                  }
                  frame True {
                    w4177 = 2 ("dimension size")
                    n2488 = Array Size(array=w4187) -> (size(s)=w4181:i32)
                    n2489 = Divide(x=w4181, y=w4177) -> (x/y=w4185:dbl)
                    n2490 = Reshape Array(w4187, w4185, w4177) -> (w4186:u64[][])
                    n2491 = Transpose 2D Array(2D array=w4186) -> (transposed array=w4184:u64[][])
                    n2492 = for {
                      tunnel: w4184 -> [w4189] mode=indexing
                      tunnel: [w4188] -> w4178 mode=indexing
                      tunnel: w4180 -> [w4190]
                      workers-P: _ -> [_]
                      n2493 = call "downsample 1D array - U64.vi"("Ave N"=w4190, "Array In"=w4189) -> ("Array Out"=w4188:u64[])  [unwired: 1 in]
                    }
                    n2494 = Transpose 2D Array(2D array=w4178) -> (transposed array=w4183:u64[][])
                    n2495 = Divide(x=w4181, y=w4180) -> (x/y=w4182:dbl)
                    n2496 = Reshape Array(w4183, w4182) -> (w4179:u64[])
                  }
                }
                n2497 = case shown="True" w4107 {
                  tunnel: w4167 -> [w4199 w4211]
                  tunnel: [w4199 w4203] -> w4163
                  tunnel: "Save ave N" -> [_ w4204]
                  tunnel: w4158 -> [_ w4202]
                  frame False {
                  }
                  frame True {
                    n2498 = Array Size(array=w4211) -> (size(s)=w4205:i32)
                    n2499 = Array Size(array=w4202) -> (size(s)=w4201:i32)
                    n2500 = Divide(x=w4205, y=w4201) -> (x/y=w4209:dbl)
                    n2501 = Reshape Array(w4211, w4209, w4201) -> (w4210:i16[][])
                    n2502 = Transpose 2D Array(2D array=w4210) -> (transposed array=w4208:i16[][])
                    n2503 = for {
                      tunnel: w4208 -> [w4214] mode=indexing
                      tunnel: [w4213] -> w4200 mode=indexing
                      tunnel: w4204 -> [w4212]
                      workers-P: _ -> [_]
                      n2504 = call "downsample 1D array - I16.vi"("Ave N"=w4212, "Array In"=w4214) -> ("Array Out"=w4213:i16[])  [unwired: 1 out]
                    }
                    n2505 = Transpose 2D Array(2D array=w4200) -> (transposed array=w4207:i16[][])
                    n2506 = Divide(x=w4205, y=w4204) -> (x/y=w4206:dbl)
                    n2507 = Reshape Array(w4207, w4206) -> (w4203:i16[])
                  }
                }
                n2508 = Index Array(array=w4129, index=1) -> (element=w4132:waveform(dbl))
                n2509 = Index Array(array=w4129, index=0) -> (element=w4134:waveform(dbl))
                n2510 = Unbundle By Name(w4132) -> ("Y"=w4136:dbl[])
                n2511 = Unbundle By Name(w4134) -> ("Y"=w4144:dbl[])
                n2512 = case "Write trap pos. data" shown="True" w4110 {
                  tunnel: w4109 -> [_ w4192]
                  tunnel: w4105 -> [_ w4191]
                  frame False {
                  }
                  frame True {
                    n2513 = Write to Binary File(file (use dialog)=w4192, data=w4191, 5:FALSE ("prepend array or string size? (T)"), 9:T24."big-endian, network order" ("byte order (0:big-endian, network order)")) -> ()  [unwired: 1 in, 4 out]
                  }
                }
                n2514 = Write to Binary File(file (use dialog)=w4170, data=w4163, 5:FALSE ("prepend array or string size? (T)"), 9:T24."big-endian, network order" ("byte order (0:big-endian, network order)")) -> ()  [unwired: 1 in, 4 out]
                n2515 = feedback #33(w4136) -> (w4138:dbl[])
                n2516 = Build Array (concatenate)(w4138, w4136) -> (w4137:dbl[])
                n2517 = Select(t=w4136, s=w4112, f=w4137) -> (s? t:f=w4122:dbl[])
                n2518 = feedback-in #33(w4122) -> ()
                n2519 = feedback #34(w4144) -> (w4157:dbl[])
                n2520 = Build Array (concatenate)(w4157, w4144) -> (w4156:dbl[])
                n2521 = Select(t=w4144, s=w4112, f=w4156) -> (s? t:f=w4131:dbl[])
                n2522 = feedback-in #34(w4131) -> ()
                n2523 = Divide(x=w4171, y=w4172) -> (x/y=w4174:dbl)
                n2524 = Multiply(x=w4174, y=100.0) -> (x*y=w4173:dbl)
                n2525 = Build Array(w4131, w4122) -> (→"Saved APD":dbl[][])
                n2526 = Array Size(array=w4131) -> (size(s)=w4149:i32)
                n2527 = Unbundle By Name(w4151) -> ("Y"=w4155:dbl[])
                n2528 = Subtract(x=w4149, y="N pts to average") -> (x-y=w4125:i32)
                n2529 = Multiply(x="N pts to average", y=u16 2) -> (x*y=w4126:u16)
                n2530 = Subtract(x=w4149, y=w4126) -> (x-y=w4124:i32)
                n2531 = feedback #35(w4155) -> (w4154:dbl[])
                n2532 = Build Array (concatenate)(w4154, w4155) -> (w4153:dbl[])
                n2533 = Select(t=w4155, s=w4112, f=w4153) -> (s? t:f=w4152:dbl[])
                "Trap Delta Graph" <- w4152
                n2534 = feedback-in #35(w4152) -> ()
                n2535 = Array Subset(array=w4131, index=w4125, length="N pts to average") -> (w4148:dbl[])
                n2536 = Array Subset(array=w4131, index=w4124, length="N pts to average") -> (w4147:dbl[])
                n2537 = Array Subset(array=w4122, index=w4125, length="N pts to average") -> (w4128:dbl[])
                n2538 = Array Subset(array=w4122, index=w4124, length="N pts to average") -> (w4127:dbl[])
                n2539 = call <vilib>:"Mean.vi"("X"=w4148) -> ("mean"=w4146:dbl)  [unwired: 1 out]
                n2540 = call <vilib>:"Mean.vi"("X"=w4128) -> ("mean"=w4121:dbl)  [unwired: 1 out]
                n2541 = call <vilib>:"Mean.vi"("X"=w4147) -> ("mean"=w4145:dbl)  [unwired: 1 out]
                n2542 = call <vilib>:"Mean.vi"("X"=w4127) -> ("mean"=w4120:dbl)  [unwired: 1 out]
                n2543 = Subtract(x=w4121, y=w4120) -> (x-y=w4111:dbl)
                "Delta Fl. 2" <- w4111
                n2544 = Subtract(x=w4146, y=w4145) -> (x-y=w4143:dbl)
                "Delta Fl. 1" <- w4143
                n2545 = Initialize Array(w4143, 1 ("dimension size")) -> (w4140:dbl[])
                n2546 = Initialize Array(w4111, 1 ("dimension size")) -> (w4117:dbl[])
                n2547 = feedback #36(w4140) -> (w4141:dbl[])
                n2548 = Build Array (concatenate)(w4141, w4140) -> (w4139:dbl[])
                n2549 = feedback #37(w4117) -> (w4118:dbl[])
                n2550 = Build Array (concatenate)(w4118, w4117) -> (w4116:dbl[])
                n2551 = Select(t=w4140, s=w4112, f=w4139) -> (s? t:f=w4115:dbl[])
                n2552 = feedback-in #36(w4115) -> ()
                n2553 = Select(t=w4117, s=w4112, f=w4116) -> (s? t:f=w4114:dbl[])
                n2554 = feedback-in #37(w4114) -> ()
                n2555 = Build Array(w4115, w4114) -> (→"Save APD Deriv":dbl[][])
              }
            }
            "Progress" <- w4088
            "Progress 2" <- w4088
          }
        }
      }
    }
    n2556 = Bundle By Name(cluster=w2784, "Green FB Ch 0"=w2783, "Green FB Ch 1"=w2782) -> (w2762:T47)
    "Green FB Signals (V)" <- w2762
    n2557 = Unbundle By Name(w2762) -> ("Green FB Ch 2"=→"Green FB Plot":dbl)
    n2558 = local read "wait to reset values"() -> (w2853:bool)
    n2559 = Not(x=w2851) -> (.not. x?=w2854:bool)
    n2560 = And(x=w2854, y=w2853) -> (x .and. y?=w2855:bool)
    n2561 = case "Part of MCL raster scanning: returns to initial positions after scan done" shown="True" w2855 {
      tunnel: w2565 -> [w3630 w3637]
      tunnel: [w3630 w3636] -> w2857
      tunnel: w2564 -> [w3629 w3635]
      tunnel: [w3629 w3634] -> w2852
      frame False {
      }
      frame True {
        w3645 = 10.0 ("y")
        w3644 = 32767.0 ("y")
        # "to return scan values\nafter a synchronous \nAOM scan"
        n2562 = local read "AO2"() -> (w3638:dbl)
        n2563 = local read "AO1"() -> (w3639:dbl)
        n2564 = local write "wait to reset values"(FALSE ("wait to reset values")) -> ()
        n2565 = Multiply(x=w3639, y=w3644) -> (x*y=w3641:dbl)
        n2566 = Multiply(x=w3638, y=w3644) -> (x*y=w3643:dbl)
        n2567 = Divide(x=w3641, y=w3645) -> (x/y=w3640:dbl)
        n2568 = Divide(x=w3643, y=w3645) -> (x/y=w3642:dbl)
        n2569 = To Word Integer(number=w3640) -> (16bit integer=w3646:i16)
        n2570 = To Word Integer(number=w3642) -> (16bit integer=w3647:i16)
        n2571 = local read "Total Counts (ticks)"() -> (w3631:u32)
        n2572 = xnode "Read/Write Control"("FPGA VI Reference In"=w3637, "error in"=w3635, "AO1"=w3646, "AO2"=w3647, "MCL count"=w3631) -> ("FPGA VI Reference Out"=w3636:T19, "error out"=w3634:errorcluster)
        n2573 = local read "Scan Range (V)\n(of steps)"() -> (w3632:dbl)
        n2574 = property on="Scan Range (V)\n(of steps)" class="DigNum (strict)"("Val(Sgnl)"=w3632) -> ()  [unwired: 2 in, 2 out]
      }
    }
    n2575 = node-c288() -> ()  [unwired: 2 out]
  }
  n2576 = node-c288(w79) -> ()  [unwired: 1 out]
  n2577 = node-c288(w81) -> ()  [unwired: 1 out]
  n2578 = node-c288(w66) -> ()  [unwired: 1 out]
  n2579 = VISA Close(VISA resource name=w70, error in (no error)=w69) -> (error out=w118:errorcluster)
  n2580 = call <vilib>:"Simple Error Handler.vi"("error in (no error)"=w118) -> ()  [unwired: 1 in, 8 out]
  n2581 = node-c288(w77) -> ()  [unwired: 1 out]
  n2582 = node-c288(w162) -> ()  [unwired: 1 out]
  n2583 = flat-sequence {
    tunnel: w256 -> [w4218]
    tunnel: w258 -> [w4219]
    tunnel: [w4217] -> w237
    tunnel: [w4216] -> w236
    tunnel: w218 -> [_]
    tunnel: w170 -> [_]
    tunnel: w83 -> [_]
    tunnel: w237 -> [w4220]
    tunnel: w236 -> [w4221]
    frame #0 {
      w4215 = FALSE ("AI to FIFO")
      n2584 = xnode "Read/Write Control"("FPGA VI Reference In"=w4219, "error in"=w4218, "AI to FIFO"=w4215, "APD to FIFO"=w4215) -> ("FPGA VI Reference Out"=w4217:T19, "error out"=w4216:errorcluster)
    }
    frame #1 {
      n2585 = xnode "Close FPGA VI Reference"("FPGA VI Reference In"=w4220, "error in"=w4221) -> ("error out"=→"error out":errorcluster)
    }
  }
